vi "Update VIPM Repo if needed.vi"(8 "error in (no error)":errorcluster, 9 "Index filename":string="index.vipr.zip", 10 "Repo URL":string="http://download.ni.com/evaluation/labview/lvtn/vipm/", 11 "Repos in":refnum<class "Repo.lvclass">[](array[class])) -> (0 "error out":errorcluster, 2 "Updated?":bool, 3 "Repos out":refnum<class "Repo.lvclass">[](array[class]))   [LabVIEW 2016, in "Packages.lvlib" / "VIPM.lvlib"]
uses:
  VIPM.lvlib
  Repo_class/Repo.lvclass
  Repo_class/Repo.lvclass/Repo.ctl
  Repo_class/Read URL.vi
  Repo_class/Read LastUpdated.vi
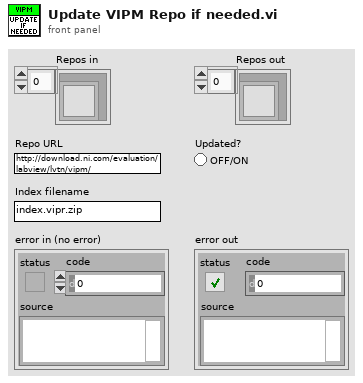
[diagram p1: front panel]
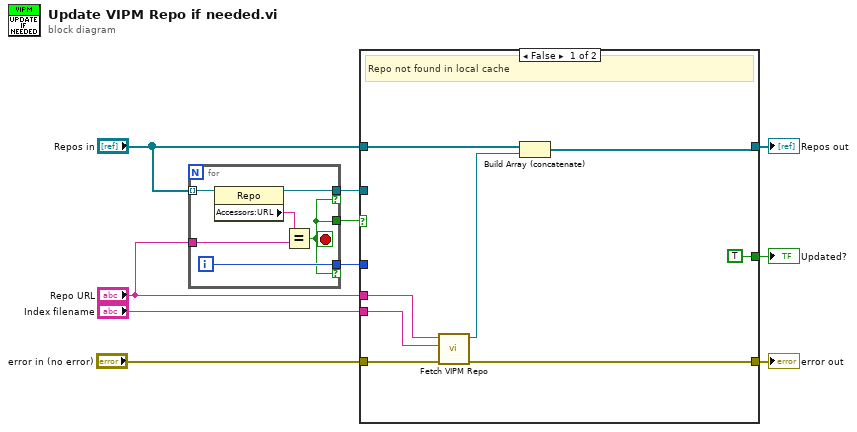
[diagram p0: block diagram]
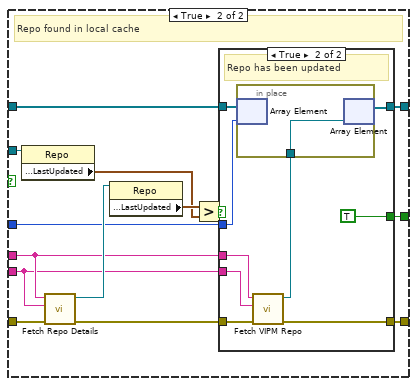
[diagram p2: hidden frame]
diagram:
  n1 = for {
    tunnel: "Repos in" -> [w16] mode=indexing
    tunnel: "Repo URL" -> [w15]
    tunnel: [w13] -> w5 if=w11
    tunnel: [w11] -> w9
    tunnel: [w12] -> w4 if=w11
    i -> [w12]
    stop <- w11 stop-if-true
    n2 = property class="Repo"(reference=w16) -> (reference out=w13:refnum<class "Repo.lvclass">, "Accessors:URL"=w14:string)  [unwired: 1 in, 1 out]
    n3 = Equal?(x=w14, y=w15) -> (x = y?=w11:bool)
  }
  n4 = case shown="False" w9 {
    tunnel: "Repos in" -> [w22 w30]
    tunnel: "error in (no error)" -> [w24 w38]
    tunnel: "Repo URL" -> [w23 w27]
    tunnel: [w20 w29] -> w3
    tunnel: [w19 w31] -> w6
    tunnel: w5 -> [_ w37]
    tunnel: w4 -> [_ w32]
    tunnel: [TRUE w26] -> w2
    tunnel: "Index filename" -> [w17 w25]
    frame False {
      # "Repo not found in local cache"
      n5 = call "Fetch VIPM Repo.vi"("error in (no error)"=w24, "Index filename"=w17, "Repo URL"=w23) -> ("error out"=w20:errorcluster, "Repo"=w21:refnum<class "Repo.lvclass">)  [unwired: 7 in]
      n6 = Build Array (concatenate)(w22, w21) -> (w19:refnum<class "Repo.lvclass">[])
    }
    frame True {
      # "Repo found in local cache"
      n7 = property class="Repo"(reference=w37) -> ("Accessors:LastUpdated"=w34:timestamp)  [unwired: 1 in, 2 out]
      n8 = call "Fetch Repo Details.vi"("error in (no error)"=w38, "Index filename"=w25, "Repo URL"=w27) -> ("error out"=w28:errorcluster, "Repo out"=w36:refnum<class "Repo.lvclass">)  [unwired: 7 in]
      n9 = property class="Repo"(reference=w36) -> ("Accessors:LastUpdated"=w35:timestamp)  [unwired: 1 in, 2 out]
      n10 = Greater?(x=w35, y=w34) -> (0:w33:bool)
      n11 = case shown="True" w33 {
        tunnel: w32 -> [_ w45]
        tunnel: [w40 w43] -> w31
        tunnel: w30 -> [w40 w46]
        tunnel: [w39 w48] -> w29
        tunnel: w28 -> [w39 w49]
        tunnel: w27 -> [_ w47]
        tunnel: [_ TRUE] -> w26
        tunnel: w25 -> [_ w41]
        frame False {
          # "Repo already up-to-date"
        }
        frame True {
          # "Repo has been updated"
          n12 = call "Fetch VIPM Repo.vi"("error in (no error)"=w49, "Index filename"=w41, "Repo URL"=w47) -> ("error out"=w48:errorcluster, "Repo"=w44:refnum<class "Repo.lvclass">)  [unwired: 7 in]
          n13 = in-place {
            in-place-border: w44 -> [w50]
            n14 = in-place-array #1(w46, w45) -> ()  [unwired: 1 out]
            n15 = in-place-array #1(w50) -> (w43:refnum<class "Repo.lvclass">[])  [unwired: 1 out]
          }
        }
      }
    }
  }
  "Repos out" <- w6
  "error out" <- w3
  "Updated?" <- w2
